vi "Save_Report_Excel.vi"(7 "Data In":string[][](array[string]), 8 "Error In":errorcluster, 10 "Headers":string[](array[string]), 11 "Report File Path In":path=path "C:/LabVIEW Projects/HLS/New Microsoft Excel Worksheet.xlsx") -> (0 "Error Out":errorcluster, 3 "Report File Path Out":path)   [LabVIEW 2014]
uses:
  <vilib>/Utility/NIReport.llb/Append Text Table to Report (wrap).vi
  <vilib>/Utility/NIReport.llb/NI_report.lvclass
  <vilib>/Utility/NIReport.llb/Excel/NI_Excel.lvclass
panel:
  # "Save Report Excel"
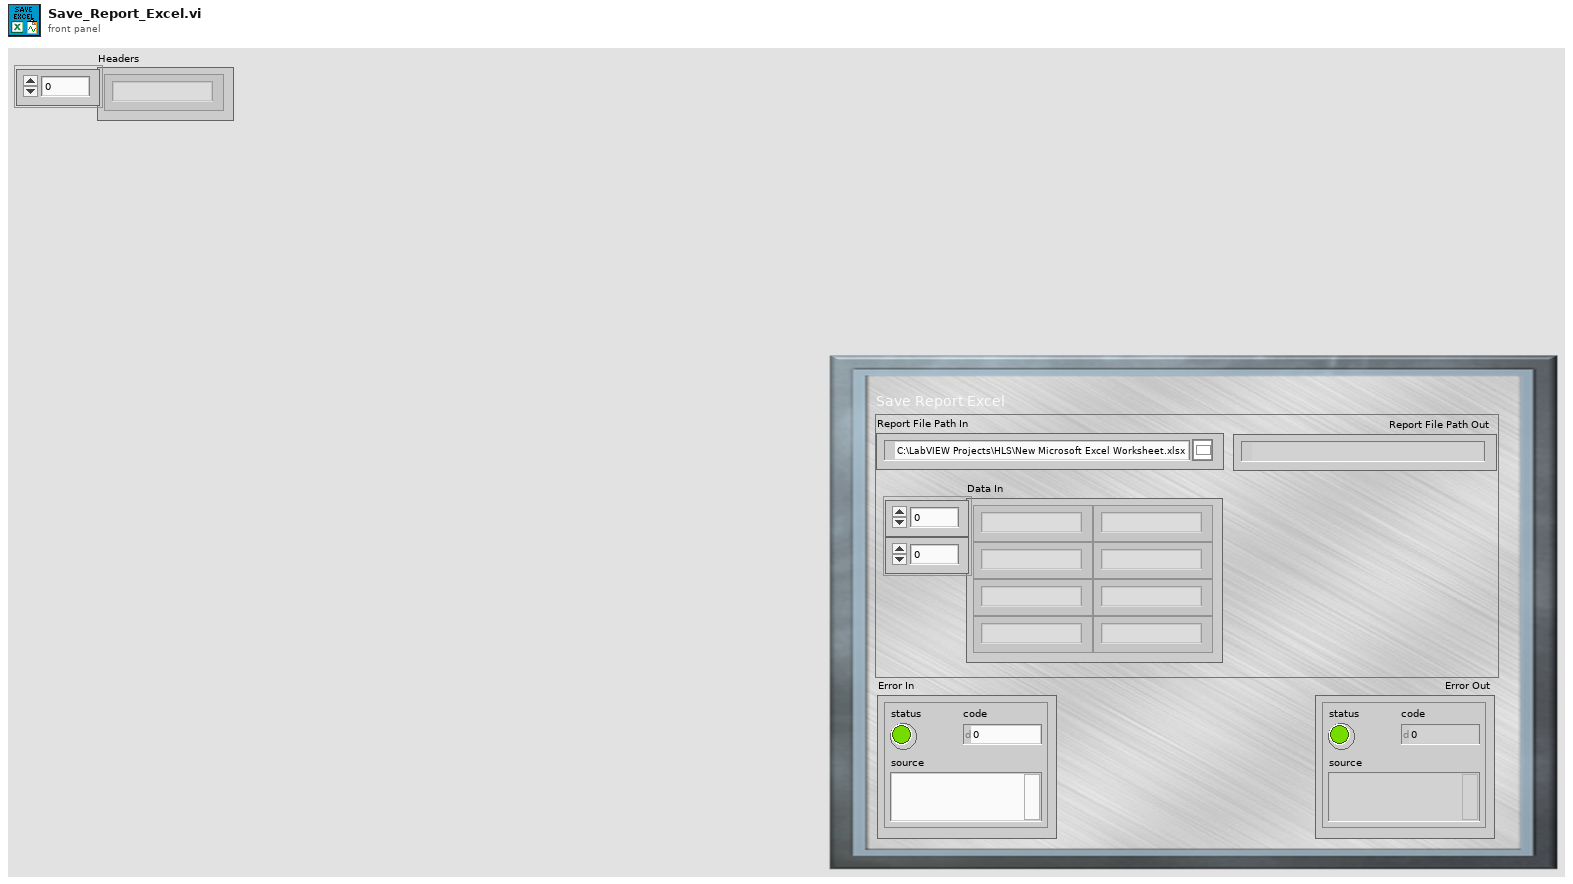
[diagram p1: front panel]
types:
  T1 = enum16{"Standard Report", "HTML", "Word", "Excel"}
  T2 = cluster{"position (Excel)":cluster{"row":i32, "column":i32}, "name (Excel)":string, "bookmark (Word)":string}
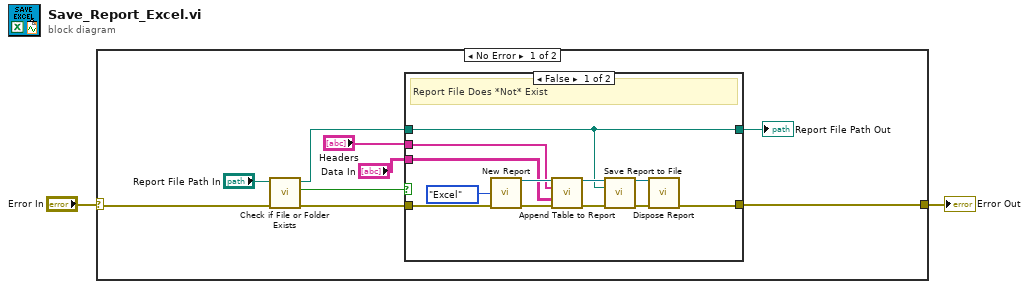
[diagram p0: block diagram]
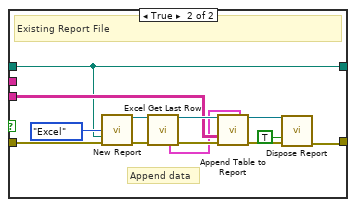
[diagram p2: hidden frame]
diagram:
  n1 = case shown="No Error" "Error In" {
    selector: "Error In" -> [w6 w37]
    tunnel: [w11 w37] -> w1
    frame No Error {
      n2 = call <vilib>:"Check if File or Folder Exists.vi"("error in (no error)"=w6, "path"="Report File Path In") -> ("error out"=w5:errorcluster, "file or folder exists?"=w9:bool, "dup path"=w4:path)  [unwired: 7 in]
      n3 = case shown="False" w9 {
        tunnel: w5 -> [w20 w35]
        tunnel: [w14 w26] -> w11
        tunnel: w4 -> [w13 w24]
        tunnel: "Data In" -> [w17 w30]
        tunnel: [w13 w24] -> w7
        tunnel: "Headers" -> [w12 _]
        frame False {
          # "Report File Does *Not* Exist"
          n4 = call <vilib>:"New Report.vi"("report type"=T1."Excel", "error in (no error)"=w20) -> ("report out"=w23:refnum<class "NI_report.lvclass">, "error out"=w21:errorcluster)  [unwired: 12 in]
          n5 = call-poly <vilib>:"Append Table to Report.vi"("report in"=w23, "column headers"=w12, "text data"=w17, "error in (no error)"=w21) -> ("report out"=w19:refnum<class "NI_report.lvclass">, "error out"=w18:errorcluster)  [unwired: 8 in, 2 out]
          n6 = call-dynamic "Save Report to File.vi"("report in"=w19, "report file path"=w13, "error in (no error)"=w18) -> ("report out"=w16:refnum<class "NI_report.lvclass">, "error out"=w15:errorcluster)  [unwired: 11 in]
          n7 = call-dynamic "Dispose Report.vi"("report in"=w16, "error in (no error)"=w15) -> ("error out"=w14:errorcluster)  [unwired: 13 in]
        }
        frame True {
          # "Append data"
          # "Existing Report File"
          n8 = call <vilib>:"New Report.vi"("report type"=T1."Excel", "template (empty)"=w24, "error in (no error)"=w35) -> ("report out"=w34:refnum<class "NI_report.lvclass">, "error out"=w33:errorcluster)  [unwired: 11 in]
          n9 = call <vilib>:"Excel Get Last Row.vi"("report in"=w34, "error in (no error)"=w33) -> ("report out"=w31:refnum<class "NI_report.lvclass">, "MS Office parameters out"=w29:T2, "error out"=w32:errorcluster)  [unwired: 11 in]
          n10 = call-poly <vilib>:"Append Table to Report.vi"("report in"=w31, "MS Office parameters"=w29, "text data"=w30, "error in (no error)"=w32) -> ("report out"=w27:refnum<class "NI_report.lvclass">, "error out"=w28:errorcluster)  [unwired: 8 in, 2 out]
          n11 = call-dynamic "Dispose Report.vi"("report in"=w27, "save changes? (F)"=TRUE, "error in (no error)"=w28) -> ("error out"=w26:errorcluster)  [unwired: 12 in]
        }
      }
      "Report File Path Out" <- w7
    }
    frame Error {
    }
  }
  "Error Out" <- w1
